vi "Set Ctrl Refnum.vi"(8 "error in (no error)":errorcluster, 10 "Ctl Refnum":refnum<vi>, 11 "Field Configuration in":refnum<class "Field Configuration.lvclass">) -> (0 "error out":errorcluster, 3 "Field Configuration out":refnum<class "Field Configuration.lvclass">)   [LabVIEW 2020, in "Basic Fields.lvlib" / "Field Configuration.lvclass"]
uses:
  Field Configuration.lvclass
  Field Configuration.lvclass/Field Configuration.ctl
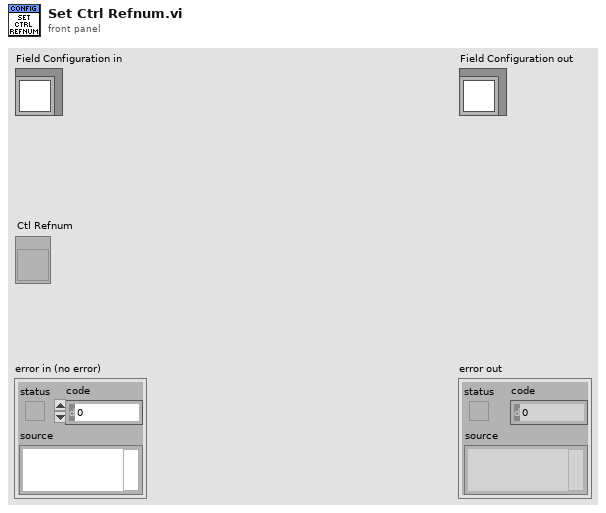
[diagram p1: front panel]
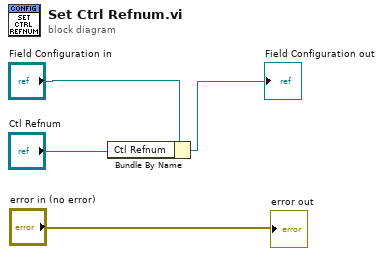
[diagram p0: block diagram]
diagram:
  n1 = Bundle By Name(cluster="Field Configuration in", "Ctl Refnum"="Ctl Refnum") -> (→"Field Configuration out":refnum<class "Field Configuration.lvclass">)
  "error out" <- "error in (no error)"
